vi "Run Tests (Path).vi"(8 "error in (no error)":errorcluster, 10 "Project or Class Path":path, 11 "Execution API In":refnum<class "Execution API.lvclass">) -> (0 "error out":errorcluster, 3 "Execution API Out":refnum<class "Execution API.lvclass">)   [LabVIEW 2020, in "Execution API.lvclass"]
doc: "Run all tests in a project or a test case at the specified path."
uses:
  Execution API.lvclass
  C:/Users/anton/Documents/GitHub/LUnit/source/Application Framework/Process Classes/Process/Process.lvclass
  Test Case/LUnit Test Case.lvclass
  Application Framework/Process Classes/Process/Process.lvclass/Process.ctl
  <vilib>/Utility/error.llb/Error Cluster From Error Code.vi
  <vilib>/ErrorRing/Error Ring.xnode
  Execution API.lvclass/Execution API.ctl
  Application Framework/Process Classes/Process/Process.lvclass
  C:/Users/anton/Documents/GitHub/LUnit/source/Framework/Execution API/Execution API.lvclass
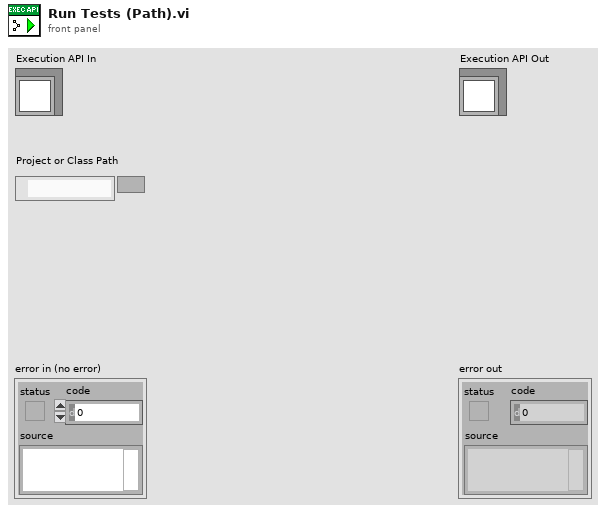
[diagram p1: front panel]
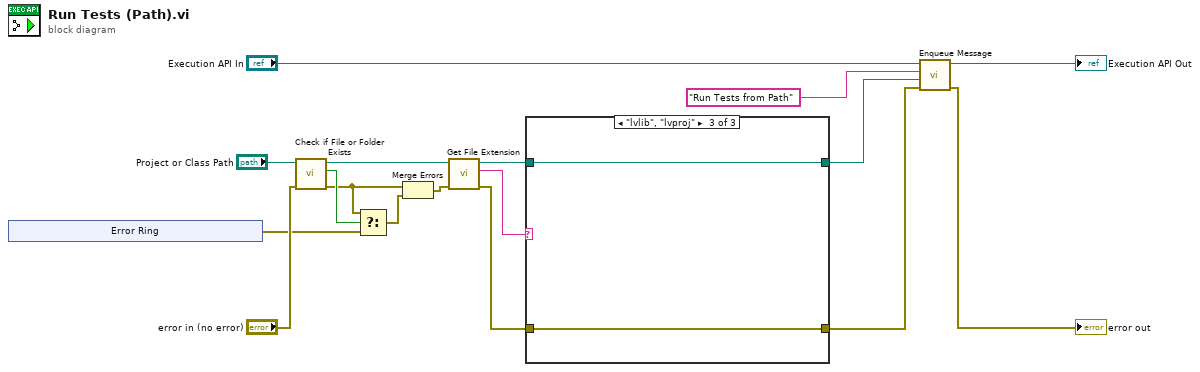
[diagram p0: block diagram]
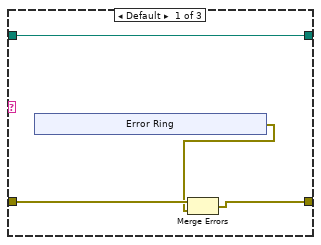
[diagram p2: hidden frame]
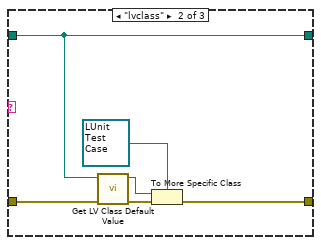
[diagram p3: hidden frame]
diagram:
  n1 = xnode "Error Ring"() -> ("error out"=w1:errorcluster)
  n2 = call <vilib>:"Check if File or Folder Exists.vi"("error in (no error)"="error in (no error)", "path"="Project or Class Path") -> ("error out"=w4:errorcluster, "file or folder exists?"=w5:bool, "dup path"=w7:path)  [unwired: 7 in]
  n3 = Select(t=w4, s=w5, f=w1) -> (s? t:f=w2:errorcluster)
  n4 = Merge Errors(w4, w2) -> (w3:errorcluster)
  n5 = call <vilib>:"Get File Extension.vi"("error in (no error)"=w3, "file"=w7) -> ("error out"=w12:errorcluster, "lowercase file extension"=w10:string, "dup file"=w13:path)  [unwired: 5 in, 2 out]
  n6 = case shown="\"lvlib\", \"lvproj\"" w10 {
    tunnel: w13 -> [w21 w26 w33]
    tunnel: w12 -> [w20 w28 w32]
    tunnel: [w19 w27 w32] -> w11
    tunnel: [w21 w26 w33] -> w9
    frame Default {
      n7 = xnode "Error Ring"() -> ("error out"=w18:errorcluster)
      n8 = Merge Errors(w20, w18) -> (w19:errorcluster)
    }
    frame "lvclass" {
      n9 = call <vilib>:"Get LV Class Default Value.vi"("error in (no error)"=w28, "class path"=w26) -> ("error out"=w31:errorcluster, "object"=w29:refnum<class>)  [unwired: 8 in]
      n10 = To More Specific Class(target class=refnum<class "LUnit Test Case.lvclass"> refnum ("LUnit Test Case.lvclass"), reference=w29, error in=w31) -> (error out=w27:errorcluster)  [unwired: 1 out]
    }
    frame "lvlib", "lvproj" {
    }
  }
  n11 = call "Enqueue Message.vi"("error in (no error)"=w11, "Message Data"=w9, "Message"="Run Tests from Path", "Process In"="Execution API In") -> ("error out"=→"error out":errorcluster, "Process Out"=→"Execution API Out":refnum<class "Execution API.lvclass">)  [unwired: 6 in]
